vi "MyPropertyClass_LV2010_Create.vi"(0 "reference in":refnum<class "MyPropertyClass_LV2010.lvclass">, 5 "error in (no error)":errorcluster) -> (14 "reference out":refnum<class "MyPropertyClass_LV2010.lvclass">, 19 "error out":errorcluster)   [LabVIEW 2020, in "MyPropertyClass_LV2010.lvclass"]
doc: "Constructor."
uses:
  MyPropertyClass_LV2010.lvclass
  C:/Program Files (x86)/National Instruments/LabVIEW 2020/vi.lib/addons/_AddQ/G#Object/G#Object.lvclass
  <vilib>/addons/_AddQ/G#Object/G#Object.lvclass
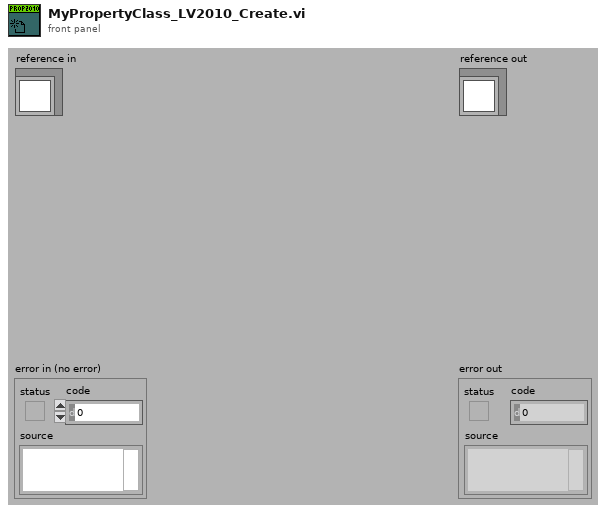
[diagram p1: front panel]
types:
  T1 = typedef "MyPropertyClass_LV2010.lvclass/ObjectAttributesRef.ctl" = refnum<data-value>
  T2 = typedef "MyPropertyClass_LV2010.lvclass/ObjectAttributes.ctl" = cluster{"MyAttribute":dbl, "Name":string}
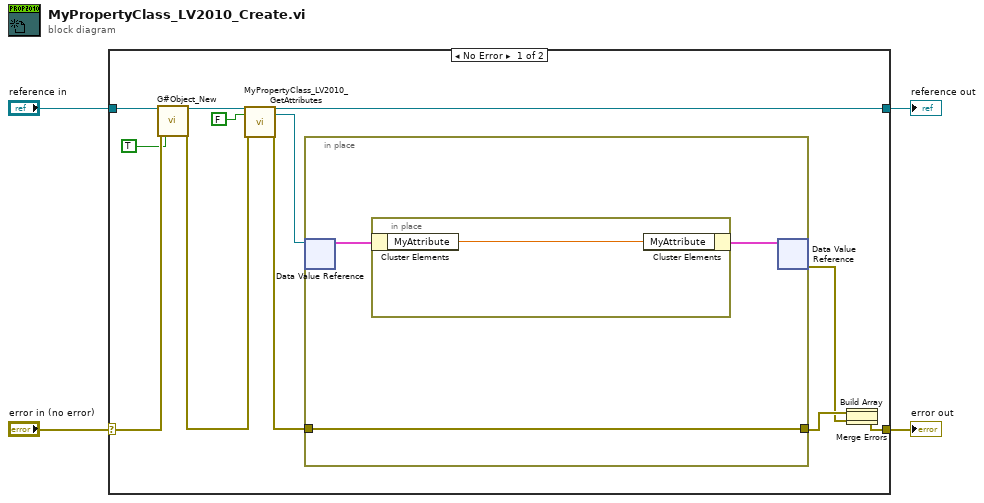
[diagram p0: block diagram]
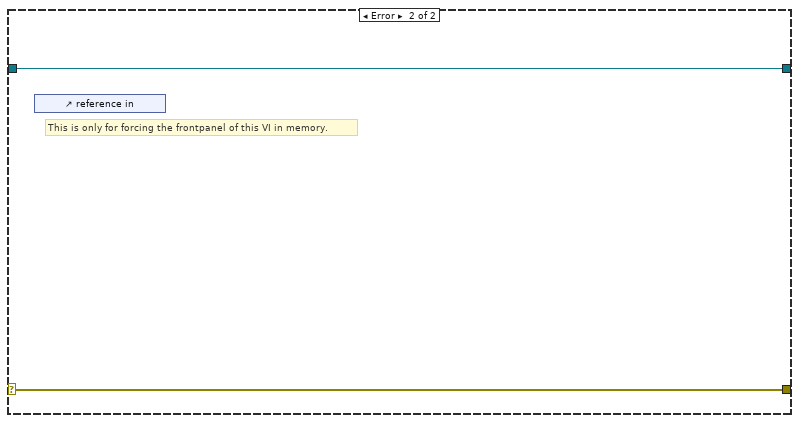
[diagram p2: hidden frame]
diagram:
  n1 = case shown="No Error" "error in (no error)" {
    selector: "error in (no error)" -> [w16 w23]
    tunnel: [w15 w23] -> w3
    tunnel: [w10 w22] -> w1
    tunnel: "reference in" -> [w17 w22]
    frame No Error {
      n2 = call <vilib>:"G#Object_New.vi"("reference in"=w17, "error in (no error)"=w16, "user counter (T)?"=TRUE ("User Counter")) -> ("reference out"=w11:refnum<class "MyPropertyClass_LV2010.lvclass">, "error out"=w9:errorcluster)  [unwired: 14 in, 1 out]
      n3 = call "MyPropertyClass_LV2010_GetAttributes.vi"("reference in"=w11, "return data? (T)"=FALSE ("return data"), "error in (no error)"=w9) -> ("reference out"=w10:refnum<class "MyPropertyClass_LV2010.lvclass">, "attributes ref"=w7:T1, "error out"=w8:errorcluster)  [unwired: 13 in, 1 out]
      n4 = in-place {
        in-place-border: w8 -> [w18]
        in-place-border: [w18] -> w13
        n5 = in-place-dvr #1(w7) -> (w19:T2)  [unwired: 1 out]
        n6 = in-place {
          n7 = in-place-cluster #2(w19) -> ("MyAttribute"=w21:dbl)
          n8 = in-place-cluster #2("MyAttribute"=w21) -> (w20:T2)
        }
        n9 = in-place-dvr #1(w20) -> (w12:errorcluster)  [unwired: 1 out]
      }
      n10 = Build Array(w13, w12) -> (w5:errorcluster[])
      n11 = Merge Errors(w5) -> (w15:errorcluster)
    }
    frame Error {
      # "This is only for forcing the frontpanel of this VI in memory."
      n12 = control-ref of="reference in"() -> ()  [unwired: 1 out]
    }
  }
  "error out" <- w3
  "reference out" <- w1
